vi "VIAn Easy Analyze.vi"(8 "error in (no error)":errorcluster, 11 "CommandLine":string[](array[string])) -> (0 "error out":errorcluster, 2 "test details":string, 3 "output to action":string)   [LabVIEW 2014]
uses:
  _lvcicd/_lvcicd_support_2014.lvlib
  <vilib>/addons/analyzer/NI_VIAnalyzerTKVIs.lvlib
panel:
  out "Total Analysis Time":dbl format="%<%M min, %S%2u sec>t"
  out "% Failed":dbl format="%.1f%%"
  out "% Passed":dbl format="%.1f%%"
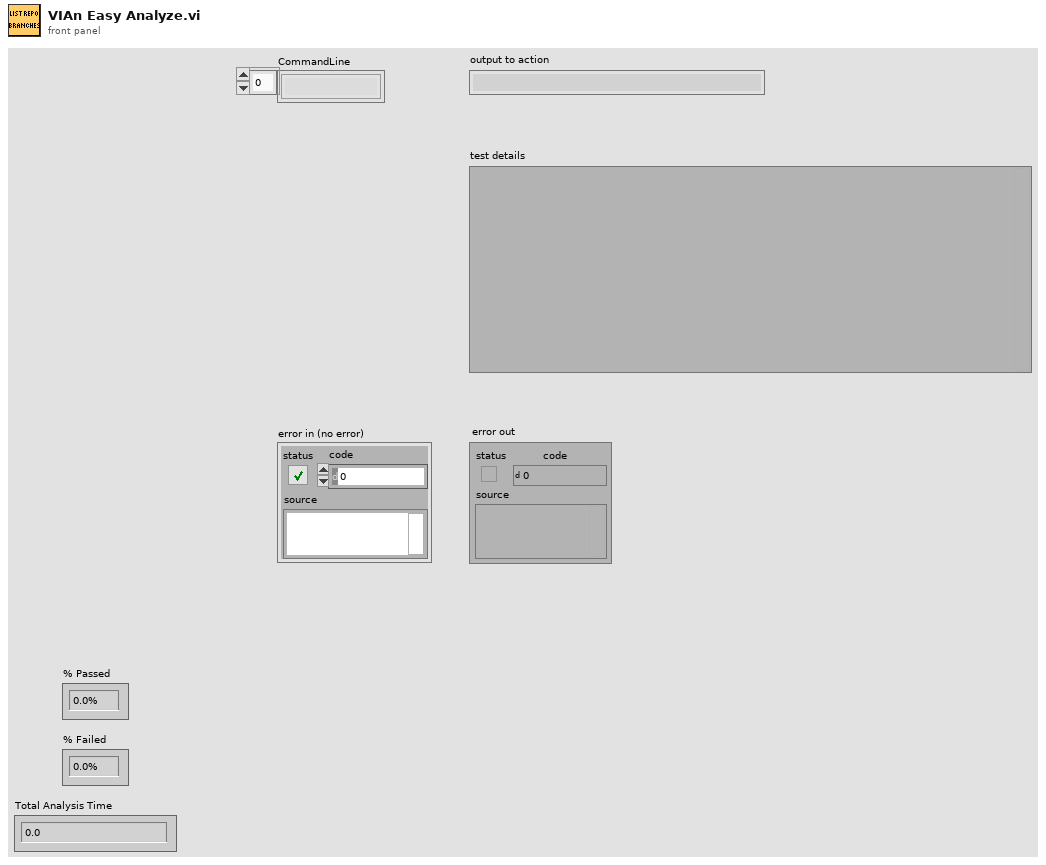
[diagram p1: front panel]
types:
  T1 = typedef "VIAnCtl Results.ctl" = cluster{"Test Name":string, "Results Data":T2[], "Status":T3, "Exceed Max Fails?":bool}
  T2 = typedef "VIAnCtl ResultsData (index).ctl" = cluster{"Result Message":string, "Ref Index":i32}
  T3 = typedef "VIAnCtl ResultStatus.ctl" = enum16{"Pass", "Fail", "Skipped", "VI not loadable", "Test not loadable", "Test not runnable", "Test error out"}
  T4 = typedef "VIAnRes Parsed Results Data (by VI).ctl" = cluster{"VI Path":path, "Pass":cluster{"row":i32, "column":i32}[], "Fail":cluster{"row":i32, "column":i32}[], "Skipped":cluster{"row":i32, "column":i32}[], "VI not loadable":cluster{"row":i32, "column":i32}[], "Test not loadable":cluster{"row":i32, "column":i32}[], "Test not runnable":cluster{"row":i32, "column":i32}[], "Test error out":cluster{"row":i32, "column":i32}[]}
  T5 = typedef "VIAnRes Parsed Results Data (by Test).ctl" = cluster{"Test Name":string, "Pass":cluster{"VI Path":path, "index":cluster{"row":i32, "column":i32}}[], "Fail":cluster{"VI Path":path, "index":cluster{"row":i32, "column":i32}}[], "Skipped":cluster{"VI Path":path, "index":cluster{"row":i32, "column":i32}}[]}
  T6 = typedef "VIAnCtl Test Config Data.ctl" = cluster{"Test Name":string, "Config Ref":refnum<vi>, "Ref Valid?":bool, "Test Ranking":T7, "Max Failures":u32, "Test Path":path, "Control Values":T8[], "Selected?":bool}
  T7 = typedef "VIAnCtl TestRanking.ctl" = u16
  T8 = typedef "VIAnCtl Config Control Value.ctl" = cluster{"Control Name":string, "Control Value":variant}
  T9 = cluster{"Raw Results":T1[][], "Parsed Results Data (by VI)":T4[], "Parsed Results Data (by Test)":T5[], "Summary Statistics":cluster{"Passed Tests":i32, "Failed Tests":i32, "Skipped Tests":i32, "VIs not loadable":i32, "Tests not loadable":i32, "Tests not runnable":i32, "Test error out":i32, "Start Time":u32, "Total Time (s)":dbl}, "Test Config Data":T6[]}
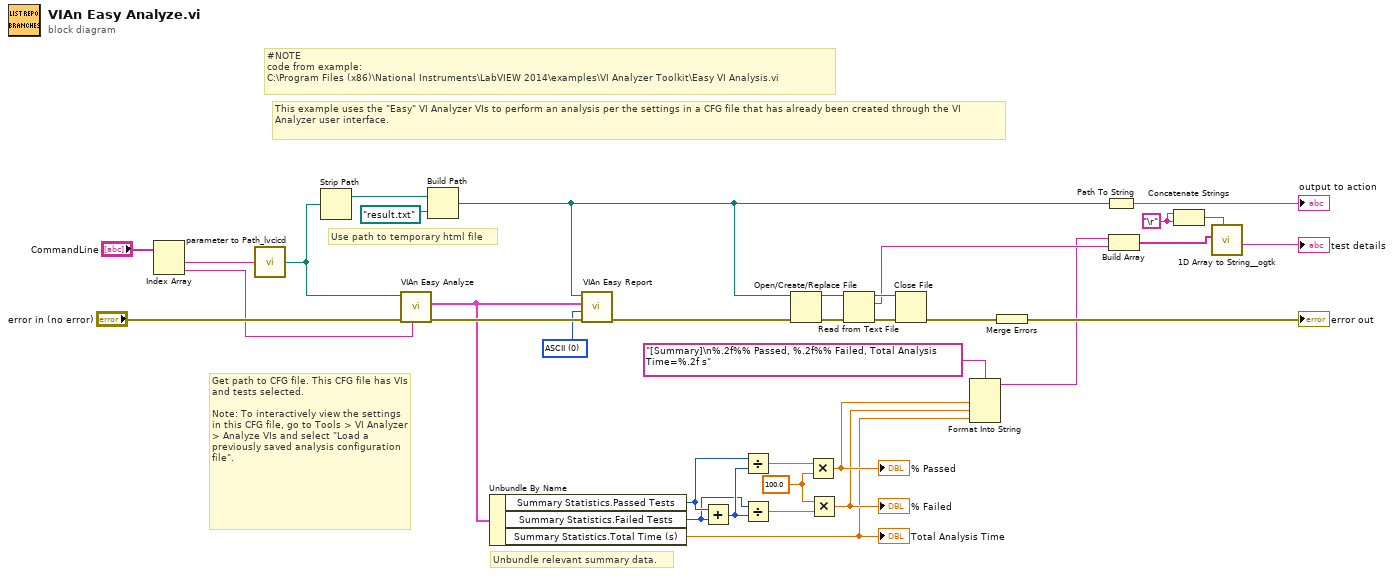
[diagram p0: block diagram]
diagram:
  w3 = "\r"
  w24 = 100.0
  w31 = u16 0 items=["ASCII", "HTML", "RSL File"] ("Report Save Type (ASCII)")
  # "#NOTE\ncode from example: \nC:\\Program Files (x86)\\National Instruments\\LabVIEW 2014\\examples\\VI Analyzer Toolkit\\Easy VI Analysis.vi"
  # "Use path to temporary html file"
  # "This example uses the \"Easy\" VI Analyzer VIs to perform an analysis per the settings in a CFG file that has already been created through the VI Analyzer user interface."
  # "Get path to CFG file. This CFG file has VIs and tests selected.\n \nNote: To interactively view the settings in this CFG file, go to Tools > VI Analyzer > Analyze VIs and select \"Load a previously saved analysis configuration file\"."
  # "Unbundle relevant summary data."
  n1 = Index Array(array="CommandLine") -> (element #1=w34:string, element #2=w9:string)  [unwired: 2 in]
  n2 = call "parameter to Path_lvcicd.vi"("String"=w34) -> ("Path"=w8:path)
  n3 = Strip Path(path=w8) -> (stripped path=w7:path)  [unwired: 1 out]
  n4 = call <vilib>:"VIAn Easy Analyze.vi"("Configuration File Password"=w9, "error in (no error)"="error in (no error)", "Analysis Target"=w8) -> ("error out"=w32:errorcluster, "Analysis Results"=w30:T9)  [unwired: 7 out]
  n5 = Build Path(base path=w7, name or relative path=path "result.txt" ("path")) -> (appended path=w6:path)
  n6 = Unbundle By Name(w30) -> ("Summary Statistics.Passed Tests"=w27:i32, "Summary Statistics.Failed Tests"=w23:i32, "Summary Statistics.Total Time (s)"=w11:dbl)
  "Total Analysis Time" <- w11
  n7 = call <vilib>:"VIAn Easy Report.vi"("error in (no error)"=w32, "Report Save Type (ASCII)"=w31, "Analysis Results"=w30, "Report Save Path"=w6) -> ("error out"=w21:errorcluster)  [unwired: 3 in, 4 out]
  n8 = Add(x=w27, y=w23) -> (x+y=w28:i32)
  n9 = Divide(x=w27, y=w28) -> (x/y=w26:dbl)
  n10 = Divide(x=w23, y=w28) -> (x/y=w25:dbl)
  n11 = Open/Create/Replace File(file path (use dialog)=w6, error in=w21) -> (refnum out=w17:refnum<file>, error out=w19:errorcluster)  [unwired: 4 in, 1 out]
  n12 = Multiply(x=w26, y=w24) -> (x*y=w13:dbl)
  "% Passed" <- w13
  n13 = Multiply(x=w24, y=w25) -> (x*y=w12:dbl)
  "% Failed" <- w12
  n14 = Read from Text File(file (use dialog)=w17, error in=w19) -> (refnum out=w16:refnum<file>, text=w15:string, error out=w18:errorcluster)  [unwired: 2 in, 1 out]
  n15 = Close File(refnum=w16, error in=w18) -> (error out=w20:errorcluster)  [unwired: 1 out]
  n16 = Format Into String(format string="[Summary]\n%.2f%% Passed, %.2f%% Failed, Total Analysis Time=%.2f s", w13, w12, w11) -> (resulting string=w10:string)  [unwired: 2 in, 1 out]
  n17 = Merge Errors(w20) -> (→"error out":errorcluster)
  n18 = Path To String(path=w6) -> (string=→"output to action":string)
  n19 = Build Array(w10, w15) -> (w2:string[])
  n20 = Concatenate Strings(w3, w3) -> (w4:string)
  n21 = call <userlib>:"1D Array to String__ogtk.vi"("delimiter (Tab)"=w4, "Array of Strings"=w2) -> ("delimited string"=→"test details":string)  [unwired: 9 in]
